vi "File Close.vi"(8 "error in (no error)":errorcluster, 11 "Logging Configuration":T1) -> (0 "error out":errorcluster)   [LabVIEW 2024]
doc: "Use the Write To Measurement File Express VI to log data to disk in a LVM file."
uses:
  Logging Configuration.ctl
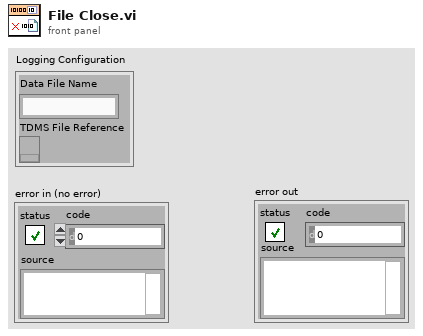
[diagram p1: front panel]
types:
  T1 = typedef "Logging Configuration.ctl" = cluster{"Data File Name":string, "TDMS File Reference":refnum<k34>}
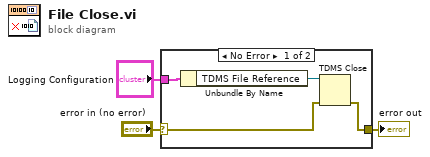
[diagram p0: block diagram]
diagram:
  n1 = case shown="No Error" "error in (no error)" {
    selector: "error in (no error)" -> [w5 w8]
    tunnel: "Logging Configuration" -> [w7 _]
    tunnel: [w6 w8] -> w2
    frame No Error {
      n2 = Unbundle By Name(w7) -> ("TDMS File Reference"=w4:refnum<k34>)
      n3 = TDMS Close(8:w5, 11:w4) -> (0:w6:errorcluster)  [unwired: 1 out]
    }
    frame Error {
    }
  }
  "error out" <- w2
